vi "Agilent_N5746A_TCP_1.vi"() -> ()   [LabVIEW 2019, in "Models of External Instruments.lvlib"]
uses:
  Models of External Instruments.lvlib
panel:
  in  "Current Amplitude":dbl
  in  "Voltage Amplitude":dbl
  out "data out":string
  out "Power data out":string
  in  "Power":bool
  in  "Enum":enum16{"Voltage", "Current"}(ring)
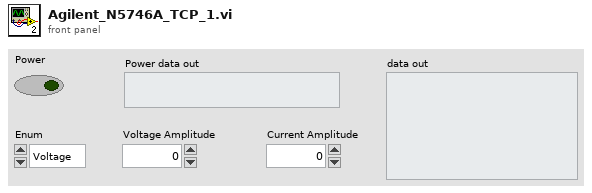
[diagram p1: front panel]
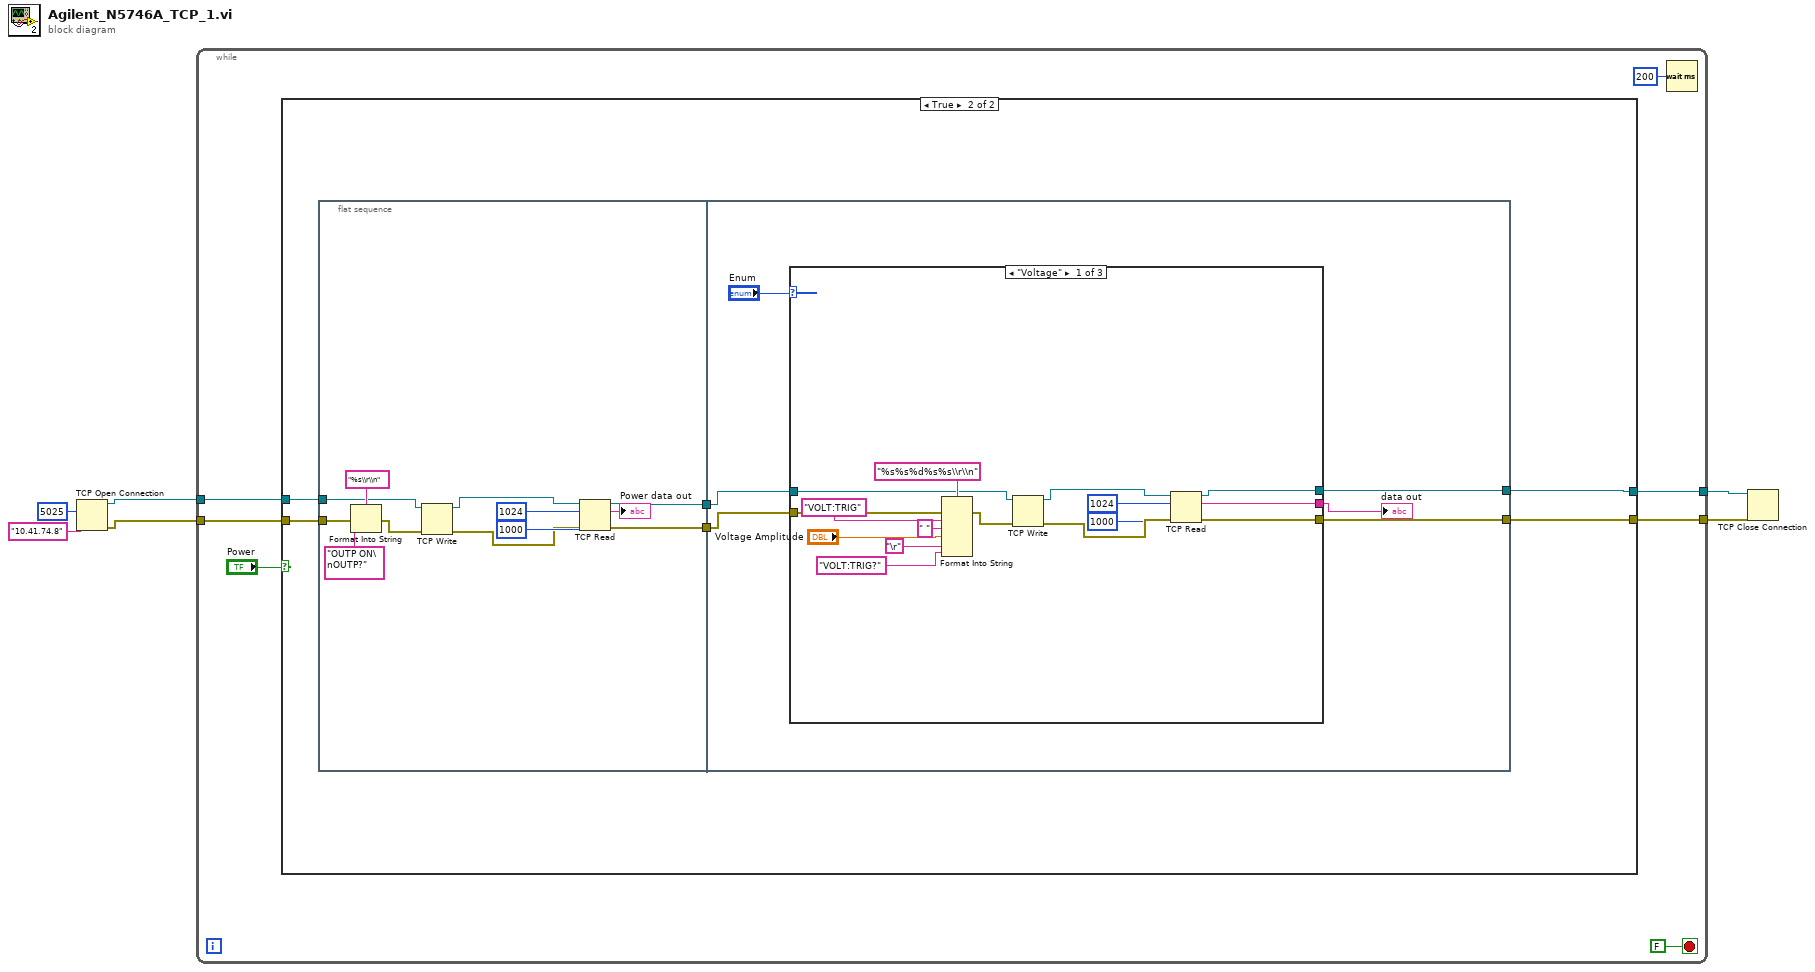
[diagram p0: block diagram]
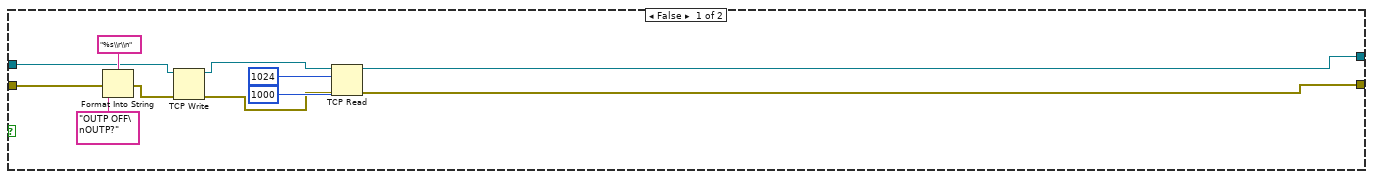
[diagram p2: hidden frame]
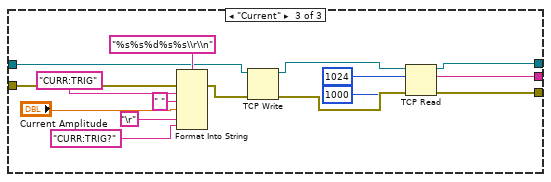
[diagram p4: hidden frame]
diagram:
  n1 = TCP Open Connection(address="10.41.74.8", remote port or service name=u16 5025) -> (connection ID=w5:refnum<k5>, error out=w6:errorcluster)  [unwired: 3 in]
  n2 = while {
    tunnel: w6 -> [w10]
    tunnel: w5 -> [w9]
    tunnel: [w8] -> w2
    tunnel: [w7] -> w1
    stop <- FALSE stop-if-true
    n3 = case shown="True" "Power" {
      tunnel: w10 -> [w16 w30]
      tunnel: w9 -> [w17 w29]
      tunnel: [w15 w26] -> w8
      tunnel: [w14 w25] -> w7
      frame False {
        n4 = Format Into String(format string="%s\\r\\n", error in=w16, "OUTP OFF\nOUTP?") -> (error out=w20:errorcluster)  [unwired: 1 in, 1 out]
        n5 = TCP Write(connection ID=w17, error in (no error)=w20) -> (connection ID out=w18:refnum<k5>, error out=w19:errorcluster)  [unwired: 2 in, 1 out]
        n6 = TCP Read(connection ID=w18, bytes to read=1024, error in (no error)=w19, 9:1000 ("timeout ms (25000)")) -> (connection ID out=w15:refnum<k5>, error out=w14:errorcluster)  [unwired: 1 in, 1 out]
      }
      frame True {
        n7 = flat-sequence {
          tunnel: w30 -> [w38]
          tunnel: w29 -> [w35]
          tunnel: [w33] -> w28
          tunnel: [w32] -> w27
          tunnel: w28 -> [w47]
          tunnel: w27 -> [w46]
          tunnel: [w45] -> w26
          tunnel: [w44] -> w25
          frame #0 {
            n8 = Format Into String(format string="%s\\r\\n", error in=w38, "OUTP ON\nOUTP?") -> (error out=w37:errorcluster)  [unwired: 1 in, 1 out]
            n9 = TCP Write(connection ID=w35, error in (no error)=w37) -> (connection ID out=w34:refnum<k5>, error out=w36:errorcluster)  [unwired: 2 in, 1 out]
            n10 = TCP Read(connection ID=w34, bytes to read=1024, error in (no error)=w36, 9:1000 ("timeout ms (25000)")) -> (connection ID out=w33:refnum<k5>, data out=→"Power data out":string, error out=w32:errorcluster)  [unwired: 1 in]
          }
          frame #1 {
            n11 = case shown="\"Voltage\"" "Enum" {
              tunnel: w47 -> [w57 w66 w72]
              tunnel: w46 -> [w56 w65 w71]
              tunnel: [w55 w66 w70] -> w45
              tunnel: [w54 w65 w68] -> w44
              tunnel: [w53 _ w69] -> w43
              frame "Voltage" {
                n12 = Format Into String(format string="%s%s%d%s%s\\r\\n", error in=w56, "VOLT:TRIG", " " ("input 2"), "Voltage Amplitude", "\r", "VOLT:TRIG?" ("input 3")) -> (error out=w62:errorcluster)  [unwired: 1 in, 1 out]
                n13 = TCP Write(connection ID=w57, error in (no error)=w62) -> (connection ID out=w64:refnum<k5>, error out=w63:errorcluster)  [unwired: 2 in, 1 out]
                n14 = TCP Read(connection ID=w64, bytes to read=1024, error in (no error)=w63, 9:1000 ("timeout ms (25000)")) -> (connection ID out=w55:refnum<k5>, data out=w53:string, error out=w54:errorcluster)  [unwired: 1 in]
              }
              frame Default {
              }
              frame "Current" {
                n15 = Format Into String(format string="%s%s%d%s%s\\r\\n", error in=w71, "CURR:TRIG", " " ("input 2"), "Current Amplitude", "\r", "CURR:TRIG?" ("input 3")) -> (error out=w80:errorcluster)  [unwired: 1 in, 1 out]
                n16 = TCP Write(connection ID=w72, error in (no error)=w80) -> (connection ID out=w82:refnum<k5>, error out=w81:errorcluster)  [unwired: 2 in, 1 out]
                n17 = TCP Read(connection ID=w82, bytes to read=1024, error in (no error)=w81, 9:1000 ("timeout ms (25000)")) -> (connection ID out=w70:refnum<k5>, data out=w69:string, error out=w68:errorcluster)  [unwired: 1 in]
              }
            }
            "data out" <- w43
          }
        }
      }
    }
    n18 = Wait (ms)(milliseconds to wait=u32 200) -> ()  [unwired: 1 out]
  }
  n19 = TCP Close Connection(connection ID=w2, error in (no error)=w1) -> ()  [unwired: 1 in, 2 out]
